vi "ComputeCellRect.vi"(8 "Column":i16=1 min=1 max=9 step=1, 9 "Line":i16=1 min=1 max=9 step=1, 10 "Cell width":i16, 11 "Border width":i16) -> (2 "Cell rect":T1)   [LabVIEW 2020]
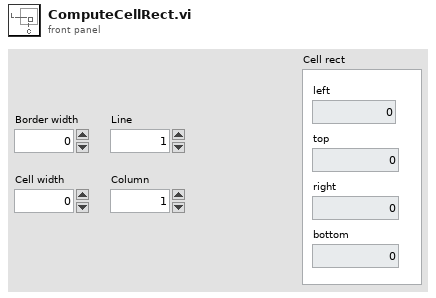
[diagram p1: front panel]
types:
  T1 = cluster{"left":i16, "top":i16, "right":i16, "bottom":u16}
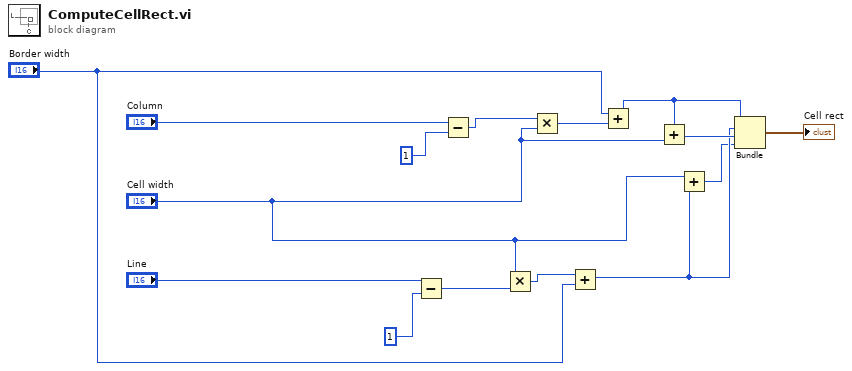
[diagram p0: block diagram]
diagram:
  n1 = Subtract(x="Line", y=1) -> (x-y=w8:i32)
  n2 = Subtract(x="Column", y=1) -> (x-y=w6:i32)
  n3 = Multiply(x="Cell width", y=w8) -> (x*y=w5:i32)
  n4 = Multiply(x=w6, y="Cell width") -> (x*y=w12:i32)
  n5 = Add(x=w5, y="Border width") -> (x+y=w2:i32)
  n6 = Add(x="Border width", y=w12) -> (x+y=w11:i32)
  n7 = Add(x=w11, y="Cell width") -> (x+y=w10:i32)
  n8 = Add(x="Cell width", y=w2) -> (x+y=w1:i32)
  n9 = Bundle(w11, w2, w10, w1) -> (→"Cell rect":cluster{i32, i32, i32, i32})  [unwired: 1 in]
